vi "Intake Controller.vi"(8 "error in":errorcluster) -> ()   [LabVIEW 2020]
doc: "This VI executes continuously carrying out the current operation and responding to updates or new operations. It will often contain the timing or control code that is difficult to place directly in TeleOp. This VI generally opens all sensors and motors and isolates the rest of the robot code from knowing how the operations are carried out."
uses:
  <vilib>/Rock Robotics/WPI/Framework/Completion Status.ctl
  Intake Setpoints.ctl
  Intake Operations.ctl
  <vilib>/Rock Robotics/WPI/ThirdParty/REV Robotics/REVLib/Typedef/Spark MAX Control Type.ctl
  <vilib>/Rock Robotics/Network Tables/NT Write Boolean.vi
panel:
  in  "Interactive Values":T1
  out "Current\nCmd":string
  in  "Buttons":cluster{"Execute Cmd":bool, "Abort Cmd":bool}
  out "Command Timing":cluster{"Start Time (ms)":u32, "Iterations":i32}
  out "Status":T3
  # "Tip: It may be helpful to observe inputs and sensor values.\nYou may also want to display tuning or debugging controls."
  # "Interactive Command: You may fill in the settings for a command\nand schedule it with the Execute button. You can observe and abort\nany command while fine tuning the code for the controller."
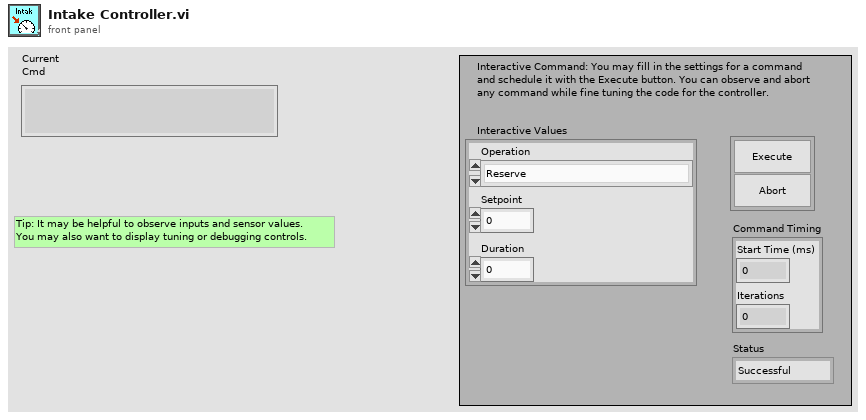
[diagram p1: front panel]
types:
  T1 = typedef "Intake Setpoints.ctl" = cluster{"Operation":T2, "Setpoint":dbl, "Duration":dbl}
  T2 = typedef "Intake Operations.ctl" = enum16{"Reserve", "Read Current", "Immediate", "Start"}
  T3 = typedef "Completion Status.ctl" = enum16{"Successful", "Aborted", "Incomplete"}
  T4 = typedef "WPI_MotorControlDeviceRef.ctl" = cluster{"DeviceStatus":errorcluster, "Type":T5, "PWM":cluster{"PWM Channel":T6, "DeadBand":T7}, "CAN":cluster{"Device Number":u8, "SetOutput VI Ref":variant, "GetOutput VI Ref":variant, "Enable VI Ref":variant, "Disable VI Ref":variant, "Data":variant}, "Invert":bool, "DIO PWM":cluster{"PWM \"Enable\" Channel":T6, "DIOChannel":T8, "PWM Rate":dbl}}
  T5 = typedef "WPI_MotorControlType.ctl" = enum16{"PWM", "CAN", "DIO PWM"}
  T6 = typedef "FPGA_DIOPWMChannel.ctl" = enum8{"PWM 0", "PWM 1", "PWM 2", "PWM 3", "PWM 4", "PWM 5", "PWM 6", "PWM 7", "PWM 8", "PWM 9", "PWM MXP 0", "PWM MXP 1", "PWM MXP 2", "PWM MXP 3", "PWM MXP 4", "PWM MXP 5", "PWM MXP 6", "PWM MXP 7", "PWM MXP 8", "PWM MXP 9", "Invalid"}
  T7 = typedef "WPI_PWMDeadband.ctl" = cluster{"Name":string, "maxPositivePwm":i32, "minPositivePwm":i32, "centerPwm":i32, "maxNegativePwm":i32, "minNegativePwm":i32, "angularRange":u16}
  T8 = typedef "FPGA_DIOChannel.ctl" = enum8{"DIO 0", "DIO 1", "DIO 2", "DIO 3", "DIO 4", "DIO 5", "DIO 6", "DIO 7", "DIO 8", "DIO 9", "DIO MXP 0", "DIO MXP 1", "DIO MXP 2", "DIO MXP 3", "DIO MXP 4", "DIO MXP 5", "DIO MXP 6", "DIO MXP 7", "DIO MXP 8", "DIO MXP 9", "DIO MXP 10", "DIO MXP 11", "DIO MXP 12", "DIO MXP 13", "DIO MXP 14", "DIO MXP 15", "SPI Port CS1", "SPI Port CS2", "SPI Port CS3", "SPI Port MISO", "SPI Port MOSI", "Invalid"}
  T9 = typedef "Command Status Info.ctl" = cluster{"Name":string, "Status":T3, "notifier out":T10}
  T10 = typedef "Completion Notifier.ctl" = refnum<notifier>
  T11 = cluster{"Current Command":T1, "Command Timing":cluster{"Start Time (ms)":u32, "Iterations":i32}, "Command Arguments":cluster{"Command Info":T9, "Description":string, "Default Command":T1, "queue out":refnum<queue>, "Subsystem Name":string}}
  T12 = typedef "Spark MAX Control Type.ctl" = enum16{"Percent VBus", "Voltage", "Velocity", "Position", "Smart Motion", "Current", "Smart Velocity"}
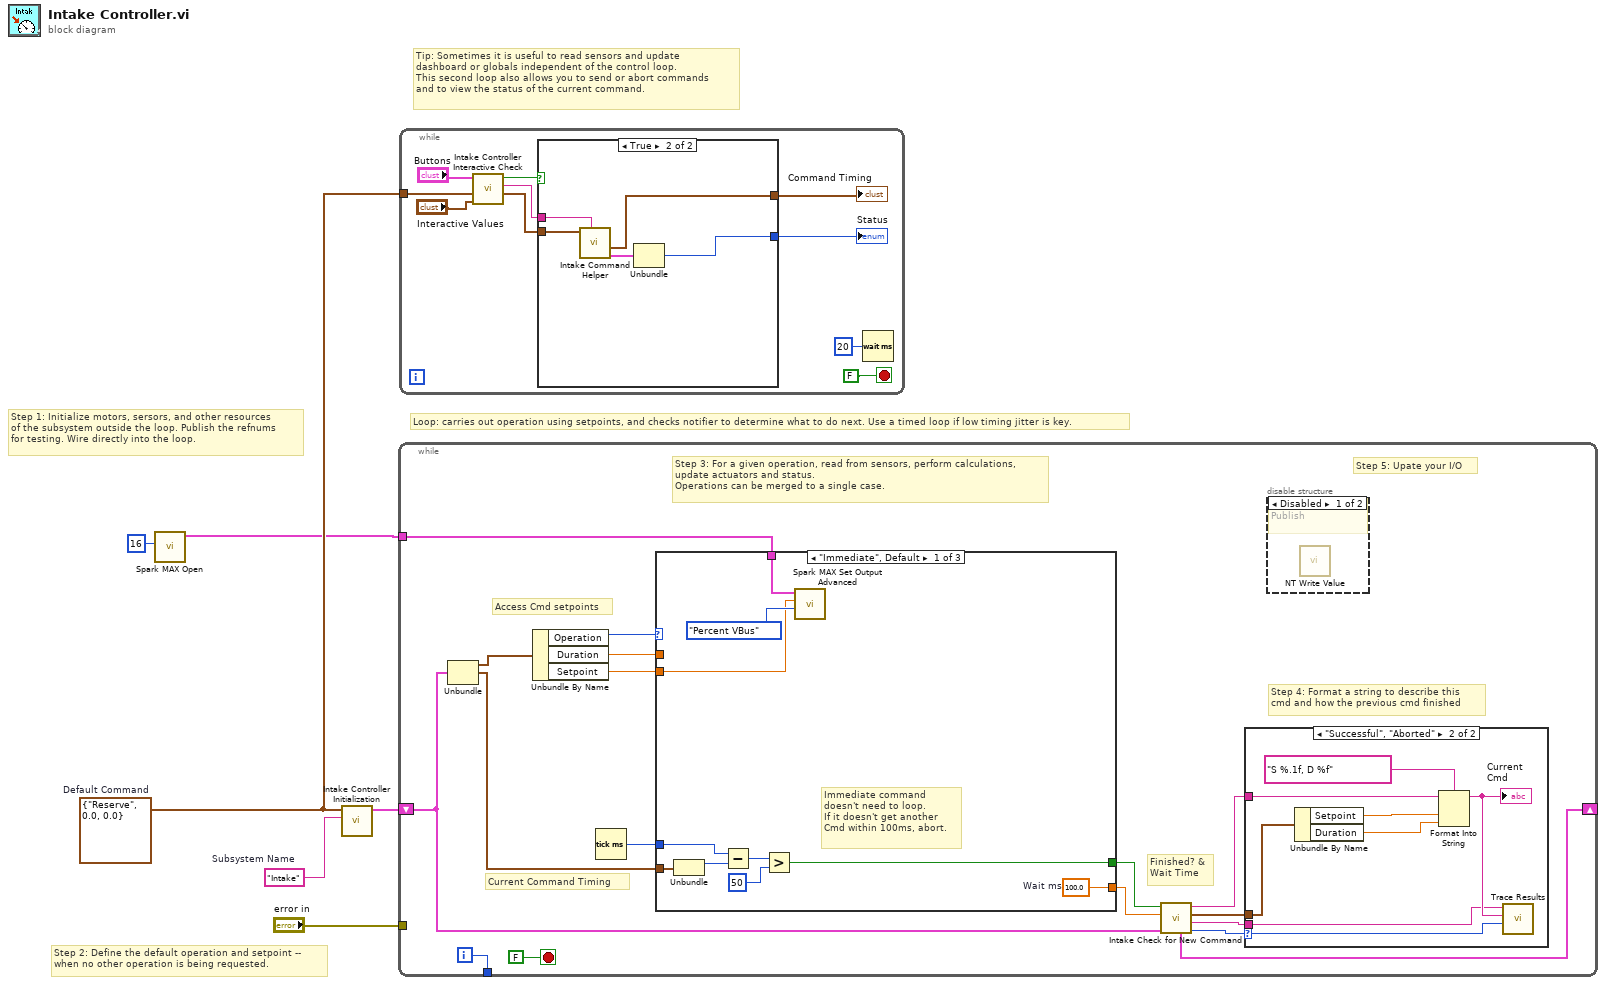
[diagram p0: block diagram]
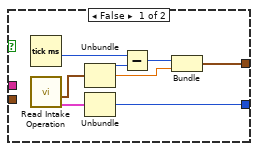
[diagram p2: hidden frame]
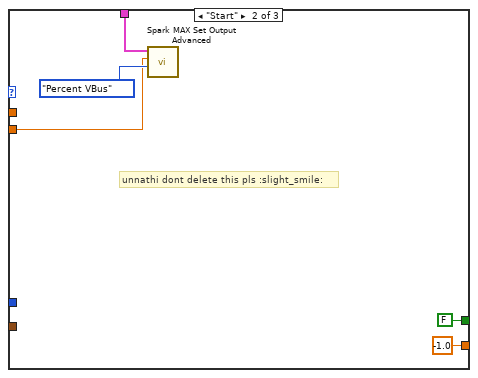
[diagram p5: hidden frame]
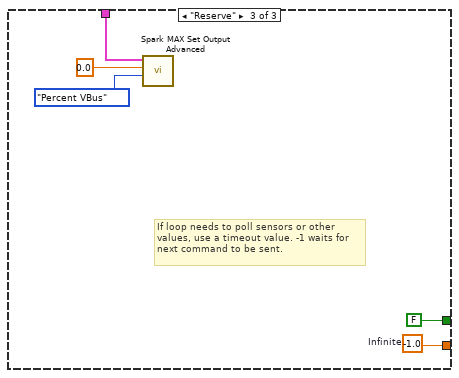
[diagram p6: hidden frame]
diagram:
  w3 = T1 {"Operation"=enum."Reserve", "Setpoint"=0.0, "Duration"=0.0}  # Default Command
  w4 = "Intake"  # Subsystem Name
  # "Tip: Sometimes it is useful to read sensors and update\ndashboard or globals independent of the control loop.\nThis second loop also allows you to send or abort commands\nand to view the status of the current command."
  # "Step 2: Define the default operation and setpoint --\nwhen no other operation is being requested."
  # "Step 1: Initialize motors, sersors, and other resources\nof the subsystem outside the loop. Publish the refnums\nfor testing. Wire directly into the loop."
  # "Loop: carries out operation using setpoints, and checks notifier to determine what to do next. Use a timed loop if low timing jitter is key."
  n1 = call <vilib>:"Spark MAX Open.vi"("Device Number"=u8 16) -> ("MotorControlDeviceRef"=w1:T4)  [unwired: 9 in, 1 out]
  n2 = call "Intake Controller Initialization.vi"("Subsystem Name"=w4, "Default Command"=w3) -> ("Current Command"=w5:T11)  [unwired: 9 in]
  n3 = while {
    shift-right: [w15] -> _
    shift-left: w5 -> [w8]
    tunnel: [w22] -> _
    tunnel: "error in" -> [_]
    tunnel: w1 -> [w7]
    i -> [w22]
    stop <- FALSE stop-if-true
    # "Step 5: Upate your I/O"
    # "Step 4: Format a string to describe this\ncmd and how the previous cmd finished"
    # "Current Command Timing"
    # "Access Cmd setpoints"
    # "Finished? &\nWait Time"
    # "Step 3: For a given operation, read from sensors, perform calculations,\nupdate actuators and status.\nOperations can be merged to a single case."
    n4 = Unbundle(w8) -> ("Current Command"=w21:T1, "Command Timing"=w17:cluster{"Start Time (ms)":u32, "Iterations":i32})  [unwired: 1 out]
    n5 = Unbundle By Name(w21) -> ("Operation"=w20:T2, "Duration"=w19:dbl, "Setpoint"=w16:dbl)
    n6 = Tick Count (ms)() -> (millisecond timer value=w18:u32)
    n7 = case shown="\"Immediate\", Default" w20 {
      tunnel: [w41 -1.0 ("Infinite") w51] -> w13
      tunnel: [w35 FALSE ("ignore previous (F)") FALSE ("ignore previous (F)")] -> w14
      tunnel: w17 -> [w37 _ _]
      tunnel: w19 -> [_ _ _]
      tunnel: w18 -> [w36 _ _]
      tunnel: w16 -> [w32 w44 _]
      tunnel: w7 -> [w34 w46 w48]
      frame "Immediate", Default {
        w41 = 100.0  # Wait ms
        # "Immediate command\ndoesn't need to loop.\nIf it doesn't get another\nCmd within 100ms, abort."
        n8 = Unbundle(w37) -> ("Start Time (ms)"=w40:u32)  [unwired: 1 out]
        n9 = Subtract(x=w36, y=w40) -> (x-y=w39:u32)
        n10 = Greater?(x=w39, y=u8 50 ("Left Motor")) -> (0:w35:bool)
        n11 = call <vilib>:"Spark MAX Set Output Advanced.vi"("Control Mode"=Spark_MAX_Control_Type."Percent VBus", "Setpoint"=w32, "MotorControlDevRef"=w34) -> ()  [unwired: 7 in, 2 out]
      }
      frame "Start" {
        # "unnathi dont delete this pls :slight_smile:"
        n12 = call <vilib>:"Spark MAX Set Output Advanced.vi"("Control Mode"=Spark_MAX_Control_Type."Percent VBus", "Setpoint"=w44, "MotorControlDevRef"=w46) -> ()  [unwired: 7 in, 2 out]
      }
      frame "Reserve" {
        w51 = -1.0  # Infinite
        # "If loop needs to poll sensors or other\nvalues, use a timeout value. -1 waits for\nnext command to be sent."
        n13 = call <vilib>:"Spark MAX Set Output Advanced.vi"("Control Mode"=Spark_MAX_Control_Type."Percent VBus", "Setpoint"=0.0, "MotorControlDevRef"=w48) -> ()  [unwired: 7 in, 2 out]
      }
    }
    n14 = call "Intake Check for New Command.vi"("Current Command"=w8, "Wait time (ms)"=w13, "Finished?"=w14) -> ("Completion"=w9:T3, "Subsystem Name"=w10:string, "Current Command"=w11:T1, "Initial Trace String"=w12:string, "NextCommand"=w15:T11)  [unwired: 4 in]
    n15 = case shown="\"Successful\", \"Aborted\"" w9 {
      selector: w9 -> [_ w31]
      tunnel: w12 -> [_ w27]
      tunnel: w11 -> [_ w28]
      tunnel: w10 -> [_ w24]
      frame "Incomplete", Default {
        # "Continuing current command"
      }
      frame "Successful", "Aborted" {
        # "Report and setup for next command"
        n16 = Unbundle By Name(w28) -> ("Setpoint"=w30:dbl, "Duration"=w25:dbl)
        n17 = Format Into String(format string="S %.1f, D %f", initial string=w27, w30, w25) -> (resulting string=w26:string)  [unwired: 1 in, 1 out]
        "Current\nCmd" <- w26
        n18 = call <vilib>:"Trace Results.vi"("Status of previous command"=w31, "Description"=w26, "Subsystem"=w24) -> ()  [unwired: 9 in]
      }
    }
    n19 = disable-structure shown="Disabled" {
      frame Disabled {
        # "Publish"
        n20 = call-poly <vilib>:"NT Write Value.vi"() -> ()  [unwired: 11 in, 1 out]
      }
      frame Enabled {
      }
    }
  }
  n21 = while {
    tunnel: w3 -> [w58]
    stop <- FALSE stop-if-true
    n22 = call "Intake Controller Interactive Check.vi"("Interactive Command in"="Interactive Values", "Default Command"=w58, "Buttons"="Buttons") -> ("Interactive Command out"=w55:T1, "Trace String"=w56:string, "Schedule"=w57:bool)  [unwired: 6 in]
    n23 = case shown="True" w57 {
      tunnel: [w69 w74] -> w54
      tunnel: w55 -> [_ w72]
      tunnel: [w65 w70] -> w53
      tunnel: w56 -> [_ w73]
      frame False {
        n24 = Tick Count (ms)() -> (millisecond timer value=w64:u32)
        n25 = call "Read Intake Operation.vi"() -> ("Command Info"=w62:T9, "SubSystem Data"=w63:T1)  [unwired: 9 in, 1 out]
        n26 = Unbundle(w63) -> ("Operation"=w68:T2, "Setpoint"=w66:dbl)  [unwired: 1 out]
        n27 = Unbundle(w62) -> ("Status"=w69:T3)  [unwired: 2 out]
        n28 = Subtract(x=w64, y=w68) -> (x-y=w67:u32)
        n29 = Bundle(w67, "Setpoint"=w66) -> (w65:cluster{u32, "Setpoint":dbl})  [unwired: 1 in]
      }
      frame True {
        n30 = call "Intake Command Helper.vi"("Description"=w73, "SubSystem Data"=w72) -> ("Command Info Out"=w71:T9, "Command Timing"=w70:cluster{"Start Time (ms)":u32, "Iterations":i32})  [unwired: 7 in, 1 out]
        n31 = Unbundle(w71) -> ("Status"=w74:T3)  [unwired: 2 out]
      }
    }
    "Status" <- w54
    "Command Timing" <- w53
    n32 = Wait (ms)(milliseconds to wait=u32 20) -> ()  [unwired: 1 out]
  }
